vi "Time elapsed.vi"(0 "Boolean in":refnum<vi>, 1 "Numeric 3":dbl, 2 "Reset Button":bool, 5 "Numeric 4":dbl, 7 "Auto Reset":bool, 11 "error in (no error)":errorcluster, 12 "Numeric in":i32) -> (3 "Present (s) 2":dbl, 4 "Present (s)":dbl, 6 "Time has Elapsed":bool, 8 "Elapsed Time Text":string, 10 "Numeric out":i32, 15 "error out":errorcluster)   [LabVIEW 2020]
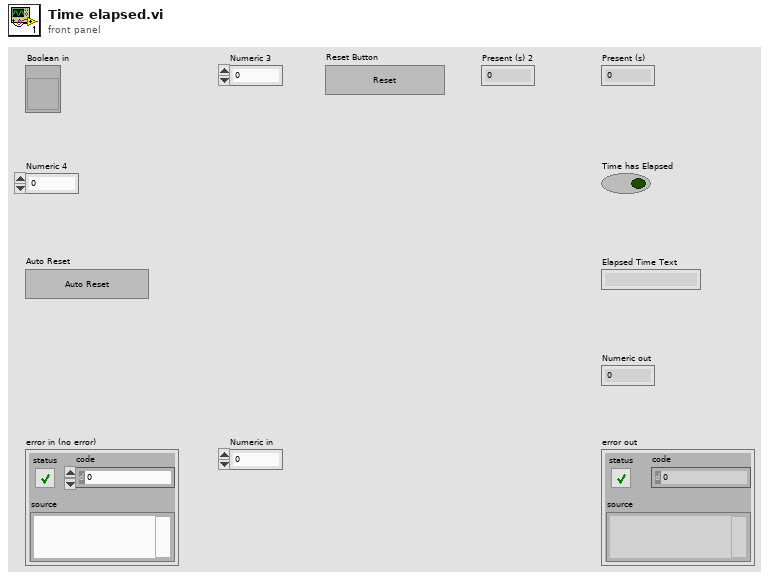
[diagram p1: front panel]
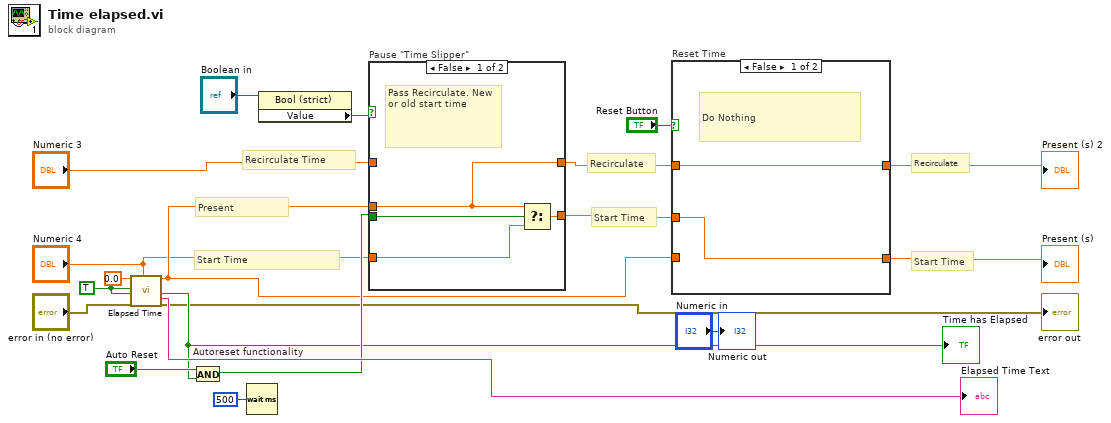
[diagram p0: block diagram]
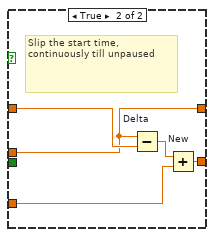
[diagram p3: hidden frame]
diagram:
  w14 = TRUE ("Reset")
  # "Present"
  # "Start Time"
  # "Recirculate Time"
  # "Recirculate"
  # "Recirculate"
  # "Start Time"
  # "Start Time"
  n1 = call "Elapsed Time"("Time Target (s)"=0.0, "Reset"=w14, "Auto Reset"=w14, "error in (no error)"="error in (no error)", "Set Start Time (s)"="Numeric 4") -> ("Present (s)"=w12:dbl, "Time has Elapsed"=w13:bool, "Elapsed Time Text"=→"Elapsed Time Text":string, "error out"=→"error out":errorcluster)  [unwired: 7 in, 4 out]
  "Time has Elapsed" <- w13
  n2 = And "Autoreset functionality"(x="Auto Reset", y=w13) -> (x .and. y?=w15:bool)
  n3 = Wait (ms)(milliseconds to wait=u32 500) -> ()  [unwired: 1 out]
  n4 = property on="Property Node" class="Bool (strict)"(reference="Boolean in") -> ("Value"=w20:bool)  [unwired: 1 in, 2 out]
  n5 = case "Pause \"Time Slipper\"" shown="False" w20 {
    tunnel: w15 -> [w24 _]
    tunnel: w12 -> [w21 w25]
    tunnel: [w23 w27] -> w10
    tunnel: "Numeric 4" -> [w22 w26]
    tunnel: [w21 w25] -> w8
    tunnel: "Numeric 3" -> [_ w28]
    frame False {
      # "Pass Recirculate. New or old start time"
      n6 = Select(t=w21, s=w24, f=w22) -> (s? t:f=w23:dbl)
    }
    frame True {
      # "Slip the start time, continuously till unpaused"
      n7 = Subtract "Delta"(x=w25, y=w28) -> (x-y=w29:dbl)
      n8 = Add "New"(x=w29, y=w26) -> (x+y=w27:dbl)
    }
  }
  n9 = case "Reset Time" shown="False" "Reset Button" {
    tunnel: [w31 w32] -> w9
    tunnel: w8 -> [w31 _]
    tunnel: [w30 w32] -> w11
    tunnel: w10 -> [w30 _]
    tunnel: w12 -> [_ w32]
    frame False {
      # "Do Nothing"
    }
    frame True {
      # "Set Both times the same"
    }
  }
  "Present (s)" <- w11
  "Present (s) 2" <- w9
  "Numeric out" <- "Numeric in"
